vi "Main.vi"() -> ()   [LabVIEW 2017]
uses:
  builds/Pojekt RubikLibrary/My Source Distribution/SingmasterMoves.ctl
  builds/Pojekt RubikLibrary/My Source Distribution/RubikLibrary.lvlib
panel:
  out "Executed Moves":T1[](array[typedef])
  in  "Execute":bool
  in  "stop":bool
  in  "Entry of Moves":T1[](array[typedef])
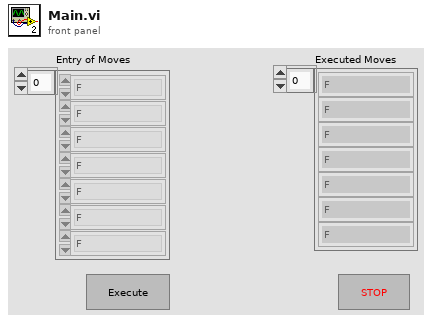
[diagram p1: front panel]
types:
  T1 = typedef "RubikLibrary.lvlib/SingmasterMoves.ctl" = enum16{"F", "B", "L", "R", "U", "D", "NO"}
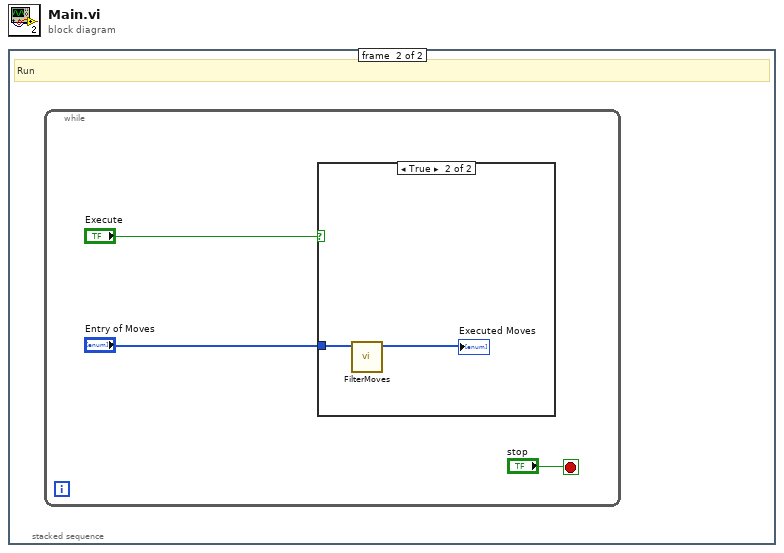
[diagram p0: block diagram]
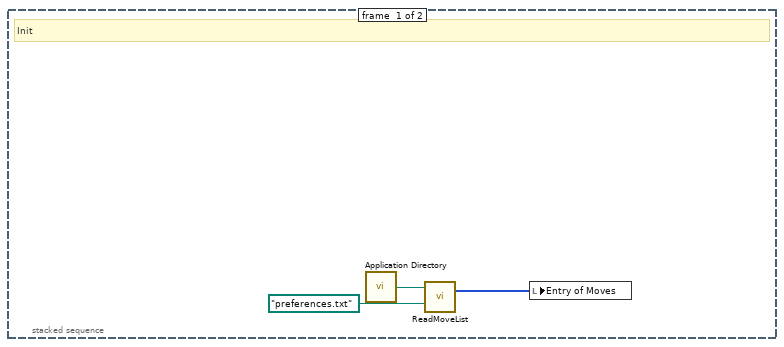
[diagram p2: hidden frame]
diagram:
  n1 = stacked-sequence {
    frame #0 {
      # "Init"
      n2 = call <vilib>:"Application Directory.vi"() -> ("Application Directory"=w2:path)
      n3 = call "ReadMoveList.vi"("default name"=path "preferences.txt", "Application Directory"=w2) -> ("Array"=w1:T1[])  [unwired: 9 in]
      n4 = local write "Entry of Moves"(w1) -> ()
    }
    frame #1 {
      # "Run"
      n5 = while {
        stop <- "stop" stop-if-true
        n6 = case shown="True" "Execute" {
          tunnel: "Entry of Moves" -> [_ w8]
          frame False {
          }
          frame True {
            n7 = call "FilterMoves.vi"("Entry of Moves"=w8) -> ("Array"=→"Executed Moves":i32[])  [unwired: 10 in]
          }
        }
      }
    }
  }
